vi "Package Info.vi"(8 "error in (no error)":errorcluster, 11 "GitPackage in":refnum<class "GitPackage.lvclass">) -> (0 "error out":errorcluster, 1 "Folder":path, 2 "Package Info":T1)   [LabVIEW 2020, in "GPack.lvlib" / "GitPackage.lvclass"]
uses:
  GitPackage.lvclass
  Package Info.ctl
  GitPackage.lvclass/GitPackage.ctl
  GPack.lvlib
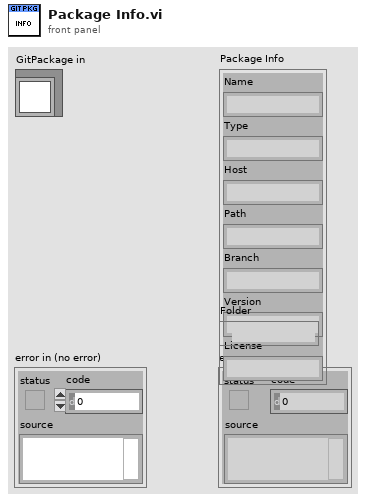
[diagram p1: front panel]
types:
  T1 = typedef "GPack.lvlib/Package Info.ctl" = cluster{"Name":string, "Type":string, "Host":string, "Path":string, "Branch":string, "Version":string, "License":string}
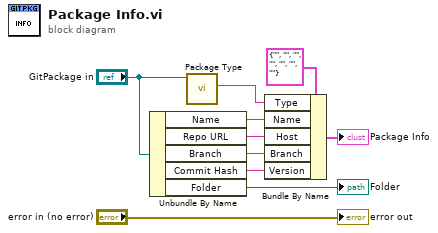
[diagram p0: block diagram]
diagram:
  n1 = Unbundle By Name("GitPackage in") -> ("Name"=w6:string, "Repo URL"=w5:string, "Branch"=w4:string, "Commit Hash"=w3:string, "Folder"=→"Folder":path)
  n2 = call-dynamic "Package Type.vi"("GitPackage in"="GitPackage in") -> ("Type"=w7:string)  [unwired: 9 in, 1 out]
  n3 = Bundle By Name(cluster=T1 {"Name"="", "Type"="", "Host"="", "Path"="", "Branch"="", "Version"="", "License"=""} ("Package Info"), "Type"=w7, "Name"=w6, "Host"=w5, "Branch"=w4, "Version"=w3) -> (→"Package Info":T1)
  "error out" <- "error in (no error)"
